vi "NavbalLabVIEW(15-5-28.vi"() -> ()   [LabVIEW 2012] (continued)
                    # "4 Planes were available:\n\nRun solver for all combinations of those 4 planes\n\nOrder:\n0) 1-1-1-1\n1) 1-0-1-1\n2) 0-1-1-1\n3) 1-1-0-1\n4) 1-0-0-1\n5) 0-1-0-1\n6) 0-0-1-1"
                    n2196 = for {
                      N: 15 -> [_]
                      tunnel: w2266 -> [w2269]
                      tunnel: w2265 -> [w2268]
                      i -> [w2270]
                      n2197 = case shown="14" w2270 {
                        tunnel: w2269 -> [w2276 w2301 w2322 w2341 w2365 w2373 w2414 w2434 w2457 w2481 w2504 w2530 w2557 w2583 w2644]
                        tunnel: w2268 -> [w2277 w2298 w2316 w2337 w2356 w2374 w2399 w2422 w2441 w2462 w2488 w2512 w2543 w2564 w2593]
                        frame 0, Default {
                          n2198 = local read "Max Iteration Count"() -> (w2275:dbl)
                          n2199 = local read "Iterative Solution?"() -> (w2274:bool)
                          n2200 = call "SolutionCalculator (SubVI) (2).vi"("Iterative?"=w2274, "Max Iteration Count"=w2275, "Base Run (matrix)"=w2277, "Response Coefficients"=w2276) -> ("Correction Phase (radians)"=w2273:T3, "RMS Residual"=w2271:dbl, "Correction Mag"=w2272:T3)  [unwired: 1 out]
                          n2201 = call-poly <vilib>:"Multiply.vi"("Real Scalar c"=180.0 ("y"), "Real Matrix A"=w2273) -> ("A * c"=w2281:T3)
                          n2202 = Divide(x=w2281, y=3.141592653589793) -> (x/y=w2279:T3)
                          n2203 = Round To Nearest(number=w2279) -> (nearest integer value=w2278:T3)
                          n2204 = local write "Final Mag 0"(w2272) -> ()
                          n2205 = local write "Resid 0"(w2271) -> ()
                          n2206 = local write "Final Phase 0"(w2278) -> ()
                        }
                        frame 1 {
                          w2302 = 2  # Plane Number
                          n2207 = Decrement(x=w2302) -> (x-1=w2299:i32)
                          n2208 = Delete From Array(array=w2301, index (col)=w2299) -> (array with subset deleted=w2297:cdb[][])  [unwired: 2 in, 1 out]
                          n2209 = local read "Max Iteration Count"() -> (w2296:dbl)
                          n2210 = local read "Iterative Solution?"() -> (w2295:bool)
                          n2211 = call "SolutionCalculator (SubVI) (2).vi"("Iterative?"=w2295, "Max Iteration Count"=w2296, "Base Run (matrix)"=w2298, "Response Coefficients"=w2297) -> ("Correction Phase (radians)"=w2293:T3, "RMS Residual"=w2283:dbl, "Correction Mag"=w2294:T3)  [unwired: 1 out]
                          n2212 = call-poly <vilib>:"Polar To Complex.vi"("Argument Q"=w2293, "Modulus r"=w2294) -> ("Complex Matrix r*e^iQ"=w2292:T15)
                          n2213 = Insert Into Array(array=w2292, index (row)=w2299, new element=cdb[] [0.0+0.0i, 0.0+0.0i] ("new element/subarray")) -> (w2284:T15)  [unwired: 1 in]
                          n2214 = call-poly <vilib>:"Complex To Polar.vi"("Complex Matrix r*e^iQ"=w2284) -> ("Modulus r"=w2291:T3, "Argument Q"=w2286:T3)
                          n2215 = call-poly <vilib>:"Multiply.vi"("Real Scalar c"=180.0 ("y"), "Real Matrix A"=w2286) -> ("A * c"=w2288:T3)
                          n2216 = local write "Resid 1"(w2283) -> ()
                          n2217 = Divide(x=w2288, y=3.141592653589793) -> (x/y=w2285:T3)
                          n2218 = Round To Nearest(number=w2285) -> (nearest integer value=w2290:T3)
                          n2219 = local write "Final Mag 1"(w2291) -> ()
                          n2220 = local write "Final Phase 1"(w2290) -> ()
                        }
                        frame 2 {
                          w2319 = 1  # Plane Number
                          n2221 = Decrement(x=w2319) -> (x-1=w2320:i32)
                          n2222 = local read "Max Iteration Count"() -> (w2314:dbl)
                          n2223 = Delete From Array(array=w2322, index (col)=w2320) -> (array with subset deleted=w2315:cdb[][])  [unwired: 2 in, 1 out]
                          n2224 = local read "Iterative Solution?"() -> (w2313:bool)
                          n2225 = call "SolutionCalculator (SubVI) (2).vi"("Iterative?"=w2313, "Max Iteration Count"=w2314, "Base Run (matrix)"=w2316, "Response Coefficients"=w2315) -> ("Correction Phase (radians)"=w2317:T3, "RMS Residual"=w2303:dbl, "Correction Mag"=w2318:T3)  [unwired: 1 out]
                          n2226 = local write "Resid 2"(w2303) -> ()
                          n2227 = call-poly <vilib>:"Polar To Complex.vi"("Argument Q"=w2317, "Modulus r"=w2318) -> ("Complex Matrix r*e^iQ"=w2312:T15)
                          n2228 = Insert Into Array(array=w2312, index (row)=w2320, new element=cdb[] [0.0+0.0i, 0.0+0.0i] ("new element/subarray")) -> (w2304:T15)  [unwired: 1 in]
                          n2229 = call-poly <vilib>:"Complex To Polar.vi"("Complex Matrix r*e^iQ"=w2304) -> ("Modulus r"=w2310:T3, "Argument Q"=w2305:T3)
                          n2230 = call-poly <vilib>:"Multiply.vi"("Real Scalar c"=180.0 ("y"), "Real Matrix A"=w2305) -> ("A * c"=w2308:T3)
                          n2231 = Divide(x=w2308, y=3.141592653589793) -> (x/y=w2306:T3)
                          n2232 = Round To Nearest(number=w2306) -> (nearest integer value=w2311:T3)
                          n2233 = local write "Final Mag  2"(w2310) -> ()
                          n2234 = local write "Final Phase 2"(w2311) -> ()
                        }
                        frame 3 {
                          w2342 = 3  # Plane Number
                          n2235 = Decrement(x=w2342) -> (x-1=w2339:i32)
                          n2236 = Delete From Array(array=w2341, index (col)=w2339) -> (array with subset deleted=w2336:cdb[][])  [unwired: 2 in, 1 out]
                          n2237 = local read "Max Iteration Count"() -> (w2335:dbl)
                          n2238 = local read "Iterative Solution?"() -> (w2334:bool)
                          n2239 = call "SolutionCalculator (SubVI) (2).vi"("Iterative?"=w2334, "Max Iteration Count"=w2335, "Base Run (matrix)"=w2337, "Response Coefficients"=w2336) -> ("Correction Phase (radians)"=w2338:T3, "RMS Residual"=w2323:dbl, "Correction Mag"=w2333:T3)  [unwired: 1 out]
                          n2240 = local write "Resid 3"(w2323) -> ()
                          n2241 = call-poly <vilib>:"Polar To Complex.vi"("Argument Q"=w2338, "Modulus r"=w2333) -> ("Complex Matrix r*e^iQ"=w2324:T15)
                          n2242 = Insert Into Array(array=w2324, index (row)=w2339, new element=cdb[] [0.0+0.0i, 0.0+0.0i] ("new element/subarray")) -> (w2325:T15)  [unwired: 1 in]
                          n2243 = call-poly <vilib>:"Complex To Polar.vi"("Complex Matrix r*e^iQ"=w2325) -> ("Modulus r"=w2326:T3, "Argument Q"=w2328:T3)
                          n2244 = call-poly <vilib>:"Multiply.vi"("Real Scalar c"=180.0 ("y"), "Real Matrix A"=w2328) -> ("A * c"=w2330:T3)
                          n2245 = Divide(x=w2330, y=3.141592653589793) -> (x/y=w2327:T3)
                          n2246 = Round To Nearest(number=w2327) -> (nearest integer value=w2332:T3)
                          n2247 = local write "Final Mag 3"(w2326) -> ()
                          n2248 = local write "Final Phase 3"(w2332) -> ()
                        }
                        frame 4 {
                          w2361 = 2  # Plane Number
                          w2366 = 3  # Plane Number
                          n2249 = local read "Max Iteration Count"() -> (w2354:dbl)
                          n2250 = local read "Iterative Solution?"() -> (w2353:bool)
                          n2251 = Decrement(x=w2366) -> (x-1=w2363:i32)
                          n2252 = Decrement(x=w2361) -> (x-1=w2360:i32)
                          n2253 = Delete From Array(array=w2365, index (col)=w2363) -> (array with subset deleted=w2362:cdb[][])  [unwired: 2 in, 1 out]
                          n2254 = Delete From Array(array=w2362, index (col)=w2360) -> (array with subset deleted=w2355:cdb[][])  [unwired: 2 in, 1 out]
                          n2255 = call "SolutionCalculator (SubVI) (2).vi"("Iterative?"=w2353, "Max Iteration Count"=w2354, "Base Run (matrix)"=w2356, "Response Coefficients"=w2355) -> ("Correction Phase (radians)"=w2357:T3, "RMS Residual"=w2343:dbl, "Correction Mag"=w2358:T3)  [unwired: 1 out]
                          n2256 = call-poly <vilib>:"Polar To Complex.vi"("Argument Q"=w2357, "Modulus r"=w2358) -> ("Complex Matrix r*e^iQ"=w2352:T15)
                          n2257 = Insert Into Array(array=w2352, index (row)=1 ("y"), new element=cdb[][] [[0.0+0.0i, 0.0+0.0i], [0.0+0.0i, 0.0+0.0i]] ("new element/subarray")) -> (w2344:T15)  [unwired: 1 in]
                          n2258 = call-poly <vilib>:"Complex To Polar.vi"("Complex Matrix r*e^iQ"=w2344) -> ("Modulus r"=w2350:T3, "Argument Q"=w2346:T3)
                          n2259 = call-poly <vilib>:"Multiply.vi"("Real Scalar c"=180.0 ("y"), "Real Matrix A"=w2346) -> ("A * c"=w2348:T3)
                          n2260 = Divide(x=w2348, y=3.141592653589793) -> (x/y=w2345:T3)
                          n2261 = Round To Nearest(number=w2345) -> (nearest integer value=w2351:T3)
                          n2262 = local write "Final Mag 4"(w2350) -> ()
                          n2263 = local write "Final Phase 4"(w2351) -> ()
                          n2264 = local write "Resid 4"(w2343) -> ()
                        }
                        frame 5 {
                          w2389 = 1  # Plane Number
                          w2392 = 3  # Plane Number
                          n2265 = local read "Max Iteration Count"() -> (w2371:dbl)
                          n2266 = local read "Iterative Solution?"() -> (w2369:bool)
                          n2267 = Decrement(x=w2392) -> (x-1=w2391:i32)
                          n2268 = Decrement(x=w2389) -> (x-1=w2388:i32)
                          n2269 = Delete From Array(array=w2373, index (col)=w2391) -> (array with subset deleted=w2390:cdb[][])  [unwired: 2 in, 1 out]
                          n2270 = Delete From Array(array=w2390, index (col)=w2388) -> (array with subset deleted=w2370:cdb[][])  [unwired: 2 in, 1 out]
                          n2271 = call "SolutionCalculator (SubVI) (2).vi"("Iterative?"=w2369, "Max Iteration Count"=w2371, "Base Run (matrix)"=w2374, "Response Coefficients"=w2370) -> ("Correction Phase (radians)"=w2375:T3, "RMS Residual"=w2367:dbl, "Correction Mag"=w2376:T3)  [unwired: 1 out]
                          n2272 = call-poly <vilib>:"Polar To Complex.vi"("Argument Q"=w2375, "Modulus r"=w2376) -> ("Complex Matrix r*e^iQ"=w2372:T15)
                          n2273 = local write "Resid 5"(w2367) -> ()
                          n2274 = Insert Into Array(array=w2372, index (row)=1, new element=cdb[] [0.0+0.0i, 0.0+0.0i] ("new element/subarray")) -> (w2385:T15)  [unwired: 1 in]
                          n2275 = Build Array (concatenate)(T15 [[0.0+0.0i]] ("array"), w2385) -> (w2368:T15)
                          n2276 = call-poly <vilib>:"Complex To Polar.vi"("Complex Matrix r*e^iQ"=w2368) -> ("Modulus r"=w2377:T3, "Argument Q"=w2380:T3)
                          n2277 = call-poly <vilib>:"Multiply.vi"("Real Scalar c"=180.0 ("y"), "Real Matrix A"=w2380) -> ("A * c"=w2382:T3)
                          n2278 = Divide(x=w2382, y=3.141592653589793) -> (x/y=w2379:T3)
                          n2279 = Round To Nearest(number=w2379) -> (nearest integer value=w2378:T3)
                          n2280 = local write "Final Mag  5"(w2377) -> ()
                          n2281 = local write "Final Phase 5"(w2378) -> ()
                        }
                        frame 6 {
                          w2409 = T15 [[0.0+0.0i]] ("array")
                          w2411 = 1  # Plane Number
                          w2415 = 2  # Plane Number
                          n2282 = local read "Max Iteration Count"() -> (w2397:dbl)
                          n2283 = local read "Iterative Solution?"() -> (w2396:bool)
                          n2284 = Decrement(x=w2415) -> (x-1=w2413:i32)
                          n2285 = Decrement(x=w2411) -> (x-1=w2410:i32)
                          n2286 = Delete From Array(array=w2414, index (col)=w2413) -> (array with subset deleted=w2412:cdb[][])  [unwired: 2 in, 1 out]
                          n2287 = Delete From Array(array=w2412, index (col)=w2410) -> (array with subset deleted=w2398:cdb[][])  [unwired: 2 in, 1 out]
                          n2288 = call "SolutionCalculator (SubVI) (2).vi"("Iterative?"=w2396, "Max Iteration Count"=w2397, "Base Run (matrix)"=w2399, "Response Coefficients"=w2398) -> ("Correction Phase (radians)"=w2400:T3, "RMS Residual"=w2393:dbl, "Correction Mag"=w2401:T3)  [unwired: 1 out]
                          n2289 = local write "Resid 6"(w2393) -> ()
                          n2290 = call-poly <vilib>:"Polar To Complex.vi"("Argument Q"=w2400, "Modulus r"=w2401) -> ("Complex Matrix r*e^iQ"=w2395:T15)
                          n2291 = Build Array (concatenate)(w2409, w2409, w2395) -> (w2394:T15)
                          n2292 = call-poly <vilib>:"Complex To Polar.vi"("Complex Matrix r*e^iQ"=w2394) -> ("Modulus r"=w2402:T3, "Argument Q"=w2405:T3)
                          n2293 = call-poly <vilib>:"Multiply.vi"("Real Scalar c"=180.0 ("y"), "Real Matrix A"=w2405) -> ("A * c"=w2407:T3)
                          n2294 = Divide(x=w2407, y=3.141592653589793) -> (x/y=w2404:T3)
                          n2295 = Round To Nearest(number=w2404) -> (nearest integer value=w2403:T3)
                          n2296 = local write "Final Phase 6"(w2403) -> ()
                          n2297 = local write "Final Mag  6"(w2402) -> ()
                        }
                        frame 7 {
                          w2435 = 4  # Plane Number
                          n2298 = local read "Max Iteration Count"() -> (w2420:dbl)
                          n2299 = local read "Iterative Solution?"() -> (w2419:bool)
                          n2300 = Decrement(x=w2435) -> (x-1=w2433:i32)
                          n2301 = Delete From Array(array=w2434, index (col)=w2433) -> (array with subset deleted=w2421:cdb[][])  [unwired: 2 in, 1 out]
                          n2302 = call "SolutionCalculator (SubVI) (2).vi"("Iterative?"=w2419, "Max Iteration Count"=w2420, "Base Run (matrix)"=w2422, "Response Coefficients"=w2421) -> ("Correction Phase (radians)"=w2423:T3, "RMS Residual"=→"Resid 7":dbl, "Correction Mag"=w2424:T3)  [unwired: 1 out]
                          n2303 = call-poly <vilib>:"Polar To Complex.vi"("Argument Q"=w2423, "Modulus r"=w2424) -> ("Complex Matrix r*e^iQ"=w2418:T15)
                          n2304 = Build Array (concatenate)(w2418, T15 [[0.0+0.0i]] ("array")) -> (w2417:T15)
                          n2305 = call-poly <vilib>:"Complex To Polar.vi"("Complex Matrix r*e^iQ"=w2417) -> ("Modulus r"=→"Final Mag  7":T3, "Argument Q"=w2427:T3)
                          n2306 = call-poly <vilib>:"Multiply.vi"("Real Scalar c"=180.0 ("y"), "Real Matrix A"=w2427) -> ("A * c"=w2429:T3)
                          n2307 = Divide(x=w2429, y=3.141592653589793) -> (x/y=w2426:T3)
                          n2308 = Round To Nearest(number=w2426) -> (nearest integer value=→"Final Phase 7":T3)
                        }
                        frame 8 {
                          w2452 = T15 [[0.0+0.0i]] ("array")
                          w2454 = 1  # Plane Number
                          w2458 = 4  # Plane Number
                          n2309 = local read "Max Iteration Count"() -> (w2440:dbl)
                          n2310 = local read "Iterative Solution?"() -> (w2439:bool)
                          n2311 = Decrement(x=w2458) -> (x-1=w2456:i32)
                          n2312 = Decrement(x=w2454) -> (x-1=w2453:i32)
                          n2313 = Delete From Array(array=w2457, index (col)=w2456) -> (array with subset deleted=w2455:cdb[][])  [unwired: 2 in, 1 out]
                          n2314 = Delete From Array(array=w2455, index (col)=w2453) -> (array with subset deleted=w2442:cdb[][])  [unwired: 2 in, 1 out]
                          n2315 = call "SolutionCalculator (SubVI) (2).vi"("Iterative?"=w2439, "Max Iteration Count"=w2440, "Base Run (matrix)"=w2441, "Response Coefficients"=w2442) -> ("Correction Phase (radians)"=w2443:T3, "RMS Residual"=→"Resid 8":dbl, "Correction Mag"=w2444:T3)  [unwired: 1 out]
                          n2316 = call-poly <vilib>:"Polar To Complex.vi"("Argument Q"=w2443, "Modulus r"=w2444) -> ("Complex Matrix r*e^iQ"=w2438:T15)
                          n2317 = Build Array (concatenate)(w2452, w2438, w2452) -> (w2437:T15)
                          n2318 = call-poly <vilib>:"Complex To Polar.vi"("Complex Matrix r*e^iQ"=w2437) -> ("Modulus r"=→"Final Mag 8":T3, "Argument Q"=w2446:T3)
                          n2319 = call-poly <vilib>:"Multiply.vi"("Real Scalar c"=180.0 ("y"), "Real Matrix A"=w2446) -> ("A * c"=w2448:T3)
                          n2320 = Divide(x=w2448, y=3.141592653589793) -> (x/y=w2445:T3)
                          n2321 = Round To Nearest(number=w2445) -> (nearest integer value=→"Final Phase 8":T3)
                        }
                        frame 9 {
                          w2478 = 2  # Plane Number
                          w2482 = 4  # Plane Number
                          n2322 = Decrement(x=w2482) -> (x-1=w2480:i32)
                          n2323 = Decrement(x=w2478) -> (x-1=w2477:i32)
                          n2324 = Delete From Array(array=w2481, index (col)=w2480) -> (array with subset deleted=w2479:cdb[][])  [unwired: 2 in, 1 out]
                          n2325 = Delete From Array(array=w2479, index (col)=w2477) -> (array with subset deleted=w2463:cdb[][])  [unwired: 2 in, 1 out]
                          n2326 = call "SolutionCalculator (SubVI) (2).vi"("Base Run (matrix)"=w2462, "Response Coefficients"=w2463) -> ("Correction Phase (radians)"=w2464:T3, "RMS Residual"=→"Resid 9":dbl, "Correction Mag"=w2465:T3)  [unwired: 2 in, 1 out]
                          n2327 = call-poly <vilib>:"Polar To Complex.vi"("Argument Q"=w2464, "Modulus r"=w2465) -> ("Complex Matrix r*e^iQ"=w2461:T15)
                          n2328 = Insert Into Array(array=w2461, index (row)=1, new element=cdb[] [0.0+0.0i, 0.0+0.0i] ("new element/subarray")) -> (w2473:T15)  [unwired: 1 in]
                          n2329 = Build Array (concatenate)(w2473, T15 [[0.0+0.0i]] ("array")) -> (w2460:T15)
                          n2330 = call-poly <vilib>:"Complex To Polar.vi"("Complex Matrix r*e^iQ"=w2460) -> ("Modulus r"=→"Final Mag 9":T3, "Argument Q"=w2467:T3)
                          n2331 = call-poly <vilib>:"Multiply.vi"("Real Scalar c"=180.0 ("y"), "Real Matrix A"=w2467) -> ("A * c"=w2469:T3)
                          n2332 = Divide(x=w2469, y=3.141592653589793) -> (x/y=w2466:T3)
                          n2333 = Round To Nearest(number=w2466) -> (nearest integer value=→"Final Phase 9":T3)
                        }
                        frame 10 {
                          w2499 = T15 [[0.0+0.0i]] ("array")
                          w2501 = 3  # Plane Number
                          w2505 = 4  # Plane Number
                          n2334 = Decrement(x=w2505) -> (x-1=w2503:i32)
                          n2335 = local read "Max Iteration Count"() -> (w2487:dbl)
                          n2336 = local read "Iterative Solution?"() -> (w2486:bool)
                          n2337 = Decrement(x=w2501) -> (x-1=w2500:i32)
                          n2338 = Delete From Array(array=w2504, index (col)=w2503) -> (array with subset deleted=w2502:cdb[][])  [unwired: 2 in, 1 out]
                          n2339 = Delete From Array(array=w2502, index (col)=w2500) -> (array with subset deleted=w2489:cdb[][])  [unwired: 2 in, 1 out]
                          n2340 = call "SolutionCalculator (SubVI) (2).vi"("Iterative?"=w2486, "Max Iteration Count"=w2487, "Base Run (matrix)"=w2488, "Response Coefficients"=w2489) -> ("Correction Phase (radians)"=w2490:T3, "RMS Residual"=→"Resid 10":dbl, "Correction Mag"=w2491:T3)  [unwired: 1 out]
                          n2341 = call-poly <vilib>:"Polar To Complex.vi"("Argument Q"=w2490, "Modulus r"=w2491) -> ("Complex Matrix r*e^iQ"=w2485:T15)
                          n2342 = Build Array (concatenate)(w2485, w2499, w2499) -> (w2484:T15)
                          n2343 = call-poly <vilib>:"Complex To Polar.vi"("Complex Matrix r*e^iQ"=w2484) -> ("Modulus r"=→"Final Mag 10":T3, "Argument Q"=w2493:T3)
                          n2344 = call-poly <vilib>:"Multiply.vi"("Real Scalar c"=180.0 ("y"), "Real Matrix A"=w2493) -> ("A * c"=w2495:T3)
                          n2345 = Divide(x=w2495, y=3.141592653589793) -> (x/y=w2492:T3)
                          n2346 = Round To Nearest(number=w2492) -> (nearest integer value=→"Final Phase 10":T3)
                        }
                        frame 11 {
                          w2523 = 2  # Plane Number
                          w2526 = T15 [[0.0+0.0i]] ("array")
                          w2522 = 3  # Plane Number
                          w2531 = 4  # Plane Number
                          n2347 = local read "Max Iteration Count"() -> (w2508:dbl)
                          n2348 = local read "Iterative Solution?"() -> (w2507:bool)
                          n2349 = Decrement(x=w2531) -> (x-1=w2529:i32)
                          n2350 = Decrement(x=w2522) -> (x-1=w2527:i32)
                          n2351 = Decrement(x=w2523) -> (x-1=w2524:i32)
                          n2352 = Delete From Array(array=w2530, index (col)=w2529) -> (array with subset deleted=w2528:cdb[][])  [unwired: 2 in, 1 out]
                          n2353 = Delete From Array(array=w2528, index (col)=w2527) -> (array with subset deleted=w2525:cdb[][])  [unwired: 2 in, 1 out]
                          n2354 = Delete From Array(array=w2525, index (col)=w2524) -> (array with subset deleted=w2511:cdb[][])  [unwired: 2 in, 1 out]
                          n2355 = call "SolutionCalculator (SubVI) (2).vi"("Iterative?"=w2507, "Max Iteration Count"=w2508, "Base Run (matrix)"=w2512, "Response Coefficients"=w2511) -> ("Correction Phase (radians)"=w2513:T3, "RMS Residual"=→"Resid 11":dbl, "Correction Mag"=w2514:T3)  [unwired: 1 out]
                          n2356 = call-poly <vilib>:"Polar To Complex.vi"("Argument Q"=w2513, "Modulus r"=w2514) -> ("Complex Matrix r*e^iQ"=w2510:T15)
                          n2357 = Build Array (concatenate)(w2510, w2526, w2526, w2526) -> (w2509:T15)
                          n2358 = call-poly <vilib>:"Complex To Polar.vi"("Complex Matrix r*e^iQ"=w2509) -> ("Modulus r"=→"Final Mag 11":T3, "Argument Q"=w2516:T3)
                          n2359 = call-poly <vilib>:"Multiply.vi"("Real Scalar c"=180.0 ("y"), "Real Matrix A"=w2516) -> ("A * c"=w2518:T3)
                          n2360 = Divide(x=w2518, y=3.141592653589793) -> (x/y=w2515:T3)
                          n2361 = Round To Nearest(number=w2515) -> (nearest integer value=→"Final Phase 11":T3)
                        }
                        frame 12 {
                          w2534 = 1  # Plane Number
                          w2554 = T15 [[0.0+0.0i]] ("array")
                          w2536 = 3  # Plane Number
                          w2538 = 4  # Plane Number
                          n2362 = Decrement(x=w2538) -> (x-1=w2537:i32)
                          n2363 = Decrement(x=w2536) -> (x-1=w2535:i32)
                          n2364 = Decrement(x=w2534) -> (x-1=w2533:i32)
                          n2365 = local read "Max Iteration Count"() -> (w2542:dbl)
                          n2366 = local read "Iterative Solution?"() -> (w2541:bool)
                          n2367 = Delete From Array(array=w2557, index (col)=w2537) -> (array with subset deleted=w2556:cdb[][])  [unwired: 2 in, 1 out]
                          n2368 = Delete From Array(array=w2556, index (col)=w2535) -> (array with subset deleted=w2555:cdb[][])  [unwired: 2 in, 1 out]
                          n2369 = Delete From Array(array=w2555, index (col)=w2533) -> (array with subset deleted=w2544:cdb[][])  [unwired: 2 in, 1 out]
                          n2370 = call "SolutionCalculator (SubVI) (2).vi"("Iterative?"=w2541, "Max Iteration Count"=w2542, "Base Run (matrix)"=w2543, "Response Coefficients"=w2544) -> ("Correction Phase (radians)"=w2545:T3, "RMS Residual"=→"Resid 12":dbl, "Correction Mag"=w2546:T3)  [unwired: 1 out]
                          n2371 = call-poly <vilib>:"Polar To Complex.vi"("Argument Q"=w2545, "Modulus r"=w2546) -> ("Complex Matrix r*e^iQ"=w2540:T15)
                          n2372 = Build Array (concatenate)(w2554, w2540, w2554, w2554) -> (w2539:T15)
                          n2373 = call-poly <vilib>:"Complex To Polar.vi"("Complex Matrix r*e^iQ"=w2539) -> ("Modulus r"=→"Final Mag 12":T3, "Argument Q"=w2548:T3)
                          n2374 = call-poly <vilib>:"Multiply.vi"("Real Scalar c"=180.0 ("y"), "Real Matrix A"=w2548) -> ("A * c"=w2550:T3)
                          n2375 = Divide(x=w2550, y=3.141592653589793) -> (x/y=w2547:T3)
                          n2376 = Round To Nearest(number=w2547) -> (nearest integer value=→"Final Phase 12":T3)
                        }
                        frame 13 {
                          w2578 = 1  # Plane Number
                          w2580 = T15 [[0.0+0.0i]] ("array")
                          w2577 = 2  # Plane Number
                          w2576 = 4  # Plane Number
                          n2377 = Decrement(x=w2576) -> (x-1=w2579:i32)
                          n2378 = Decrement(x=w2577) -> (x-1=w2575:i32)
                          n2379 = Decrement(x=w2578) -> (x-1=w2574:i32)
                          n2380 = Delete From Array(array=w2583, index (col)=w2579) -> (array with subset deleted=w2582:cdb[][])  [unwired: 2 in, 1 out]
                          n2381 = Delete From Array(array=w2582, index (col)=w2575) -> (array with subset deleted=w2581:cdb[][])  [unwired: 2 in, 1 out]
                          n2382 = local read "Max Iteration Count"() -> (w2562:dbl)
                          n2383 = local read "Iterative Solution?"() -> (w2561:bool)
                          n2384 = Delete From Array(array=w2581, index (col)=w2574) -> (array with subset deleted=w2563:cdb[][])  [unwired: 2 in, 1 out]
                          n2385 = call "SolutionCalculator (SubVI) (2).vi"("Iterative?"=w2561, "Max Iteration Count"=w2562, "Base Run (matrix)"=w2564, "Response Coefficients"=w2563) -> ("Correction Phase (radians)"=w2565:T3, "RMS Residual"=→"Resid 13":dbl, "Correction Mag"=w2566:T3)  [unwired: 1 out]
                          n2386 = call-poly <vilib>:"Polar To Complex.vi"("Argument Q"=w2565, "Modulus r"=w2566) -> ("Complex Matrix r*e^iQ"=w2560:T15)
                          n2387 = Build Array (concatenate)(w2580, w2580, w2560, w2580) -> (w2559:T15)
                          n2388 = call-poly <vilib>:"Complex To Polar.vi"("Complex Matrix r*e^iQ"=w2559) -> ("Modulus r"=→"Final Mag 13":T3, "Argument Q"=w2568:T3)
                          n2389 = call-poly <vilib>:"Multiply.vi"("Real Scalar c"=180.0 ("y"), "Real Matrix A"=w2568) -> ("A * c"=w2570:T3)
                          n2390 = Divide(x=w2570, y=3.141592653589793) -> (x/y=w2567:T3)
                          n2391 = Round To Nearest(number=w2567) -> (nearest integer value=→"Final Phase 13":T3)
                        }
                        frame 14 {
                          w2604 = 1  # Plane Number
                          w2641 = T15 [[0.0+0.0i]] ("array")
                          w2605 = 2  # Plane Number
                          w2606 = 3  # Plane Number
                          n2392 = local read "Max Iteration Count"() -> (w2591:dbl)
                          n2393 = local read "Iterative Solution?"() -> (w2590:bool)
                          n2394 = Decrement(x=w2606) -> (x-1=w2587:i32)
                          n2395 = Decrement(x=w2605) -> (x-1=w2602:i32)
                          n2396 = Decrement(x=w2604) -> (x-1=w2603:i32)
                          n2397 = Delete From Array(array=w2644, index (col)=w2587) -> (array with subset deleted=w2643:cdb[][])  [unwired: 2 in, 1 out]
                          n2398 = Delete From Array(array=w2643, index (col)=w2602) -> (array with subset deleted=w2642:cdb[][])  [unwired: 2 in, 1 out]
                          n2399 = Delete From Array(array=w2642, index (col)=w2603) -> (array with subset deleted=w2592:cdb[][])  [unwired: 2 in, 1 out]
                          n2400 = call "SolutionCalculator (SubVI) (2).vi"("Iterative?"=w2590, "Max Iteration Count"=w2591, "Base Run (matrix)"=w2593, "Response Coefficients"=w2592) -> ("Correction Phase (radians)"=w2594:T3, "RMS Residual"=w2586:dbl, "Correction Mag"=w2595:T3)  [unwired: 1 out]
                          "Resid 14" <- w2586
                          n2401 = call-poly <vilib>:"Polar To Complex.vi"("Argument Q"=w2594, "Modulus r"=w2595) -> ("Complex Matrix r*e^iQ"=w2589:T15)
                          n2402 = Build Array (concatenate)(w2641, w2641, w2641, w2589) -> (w2588:T15)
                          n2403 = local read "Final Mag 0"() -> (w2620:T3)
                          n2404 = local read "Final Mag  2"() -> (w2617:T3)
                          n2405 = local read "Final Mag  5"() -> (w2614:T3)
                          n2406 = local read "Final Mag  6"() -> (w2624:T3)
                          n2407 = local read "Final Mag  7"() -> (w2625:T3)
                          n2408 = local read "Final Mag 9"() -> (w2627:T3)
                          n2409 = local read "Final Mag 1"() -> (w2621:T3)
                          n2410 = local read "Final Mag 3"() -> (w2616:T3)
                          n2411 = local read "Final Mag 4"() -> (w2615:T3)
                          n2412 = local read "Final Mag 8"() -> (w2626:T3)
                          n2413 = local read "Final Mag 10"() -> (w2628:T3)
                          n2414 = local read "Final Mag 11"() -> (w2629:T3)
                          n2415 = local read "Final Mag 12"() -> (w2630:T3)
                          n2416 = local read "Final Mag 13"() -> (w2631:T3)
                          n2417 = call-poly <vilib>:"Complex To Polar.vi"("Complex Matrix r*e^iQ"=w2588) -> ("Modulus r"=w2609:T3, "Argument Q"=w2597:T3)
                          "Final Mag 14" <- w2609
                          n2418 = call-poly <vilib>:"Multiply.vi"("Real Scalar c"=180.0 ("y"), "Real Matrix A"=w2597) -> ("A * c"=w2599:T3)
                          n2419 = Divide(x=w2599, y=3.141592653589793) -> (x/y=w2596:T3)
                          n2420 = Build Array (concatenate)(w2620, w2621, w2617, w2616, w2615, w2614, w2624, w2625, w2626, w2627, w2628, w2629, w2630, w2631, w2609) -> (w2608:T3)
                          n2421 = Round To Nearest(number=w2596) -> (nearest integer value=→"Final Phase 14":T3)
                          n2422 = local read "Resid 0"() -> (w2618:dbl)
                          n2423 = local read "Resid 1"() -> (w2619:dbl)
                          n2424 = local read "Resid 2"() -> (w2613:dbl)
                          n2425 = local read "Resid 3"() -> (w2612:dbl)
                          n2426 = local read "Resid 4"() -> (w2611:dbl)
                          n2427 = local read "Resid 5"() -> (w2610:dbl)
                          n2428 = local read "Resid 6"() -> (w2632:dbl)
                          n2429 = local read "Resid 7"() -> (w2633:dbl)
                          n2430 = local read "Resid 8"() -> (w2634:dbl)
                          n2431 = local read "Resid 9"() -> (w2635:dbl)
                          n2432 = local read "Resid 10"() -> (w2636:dbl)
                          n2433 = local read "Resid 11"() -> (w2637:dbl)
                          n2434 = local read "Resid 12"() -> (w2638:dbl)
                          n2435 = local read "Resid 13"() -> (w2639:dbl)
                          n2436 = Transpose 2D Array(2D array=w2608) -> (transposed array=w2607:T3)
                          n2437 = Build Array(w2618, w2619, w2613, w2612, w2611, w2610, w2632, w2633, w2634, w2635, w2636, w2637, w2638, w2639, w2586) -> (w2640:T3)
                          n2438 = Build Array (concatenate)(w2607, w2640) -> (w2623:T3)
                          n2439 = Number To Fractional String(number=w2623, precision (6)=i16 3) -> (F-format string=w2585:string[][])  [unwired: 2 in]
                          n2440 = for {
                            tunnel: w2585 -> [w2646] mode=indexing
                            tunnel: [w2645] -> w2584 mode=indexing
                            n2441 = for {
                              tunnel: w2646 -> [w2647] mode=indexing
                              tunnel: [w2648] -> w2645 mode=indexing
                              n2442 = Equal?(x="0.000", y=w2647) -> (x = y?=w2649:bool)
                              n2443 = case shown="False" w2649 {
                                tunnel: [w2651 ""] -> w2648
                                tunnel: w2647 -> [w2651 _]
                                frame False {
                                }
                                frame True {
                                }
                              }
                            }
                          }
                          n2444 = property on="Solution Options" class="MCListbox (strict)"("ItemNames"=w2584) -> ()  [unwired: 2 in, 2 out]
                        }
                      }
                    }
                  }
                }
              }
            }
          }
        }
        n2445 = case "Begin Weight Splitting Procedure:\n\nProcess is to use a binary search algorithm to most closely match the  \"ideal vector\". If we use brute force, solution\ncomplexity is about N^2, or about 2e8 combinations, versus the binary search, which is NlogN, or 6e4 combinations \n\nProcess also checks to see if current hole is occupied in that plane, and will alter vector combinations which use that hole\nso that they are not selected as the best combination" shown="True" "Split Weights" {
          tunnel: "Degrees" -> [_ w2657]
          tunnel: "Ideal Weight" -> [_ w2659]
          tunnel: w634 -> [_ w2658]
          frame False {
            # "Useful to check here, but I didnt store any code inside.\n\n-Belding"
          }
          frame True {
            w2660 = u32 2771455
            # "Generate ideal  complex vector"
            # "4 planes"
            # "get number of \nholes"
            n2446 = Divide(x=w2657, y=180.0 ("x")) -> (x/y=w2664:T3)
            n2447 = for "Clear Prediction highlights" {
              N: 50 -> [_]
              i -> [w2672]
              n2448 = Bundle(w2672, "Column"=3) -> (w2671:cluster{i32, "Column":i32})  [unwired: 1 in]
              n2449 = property on="Prediction Results" class="MCListbox (strict)"("ActiveCell"=w2671) -> ()  [unwired: 2 in, 2 out]
              n2450 = property on="Prediction Results" class="MCListbox (strict)"("CellBG"=u32 16777215) -> ()  [unwired: 2 in, 2 out]
            }
            n2451 = property on="Aft Turbine Balance Plane Split Options" class="MCListbox (strict)"("SelColor"=w2660) -> ()  [unwired: 2 in, 2 out]
            n2452 = property on="Fwd Turbine Balance Plane Split Options" class="MCListbox (strict)"("SelColor"=w2660) -> ()  [unwired: 2 in, 2 out]
            n2453 = case shown="\"Port\"" w2658 {
              tunnel: ["Existing Plane Wts Stbd" "Existing Plane Wts Port"] -> w2653
              frame "Starboard", Default {
              }
              frame "Port" {
              }
            }
            n2454 = property on="Aft Generator Balance Plane Split Options" class="MCListbox (strict)"("SelColor"=w2660) -> ()  [unwired: 2 in, 2 out]
            n2455 = property on="Fwd Generator Balance Plane Split Options" class="MCListbox (strict)"("SelColor"=w2660) -> ()  [unwired: 2 in, 2 out]
            n2456 = call-poly <vilib>:"Multiply.vi"("Real Matrix A"=w2664, "Real Scalar c"=3.141592653589793) -> ("c * A"=w2665:T3)
            n2457 = call-poly <vilib>:"Multiply.vi"("Real Matrix A"="Divisions in\nEach Plane", "Real Scalar c"="Holes/Division") -> ("c * A"=w2662:T3)
            n2458 = call-poly <vilib>:"Polar To Complex.vi"("Argument Q"=w2665, "Modulus r"=w2659) -> ("Complex Matrix r*e^iQ"=w2663:T15)
            n2459 = Matrix Size(0:w2659) -> (1:w2668:i32)  [unwired: 1 out]
            n2460 = for {
              N: w2668 -> [_]
              tunnel: w2659 -> [w2700] mode=indexing
              tunnel: w2663 -> [w2696] mode=indexing
              tunnel: w2662 -> [w2697] mode=indexing
              tunnel: w2657 -> [w2698] mode=indexing
              tunnel: "Divisions in\nEach Plane" -> [w2694] mode=indexing
              tunnel: [w2689] -> w2654 mode=indexing
              tunnel: w2653 -> [w2686]
              i -> [w2688]
              # "Places data into the listbox of split options"
              n2461 = Index Array(array=w2700, index=0) -> (element=w2676:dbl)
              n2462 = Not Equal To 0?(x=w2676) -> (x != 0?=w2675:bool)
              n2463 = case shown="True" w2675 {
                tunnel: [w2707 w2803] -> w2701
                tunnel: [w2707 w2802] -> w2699
                tunnel: w2698 -> [_ w2800]
                tunnel: w2697 -> [_ w2799]
                tunnel: w2696 -> [_ w2787]
                tunnel: [w2707 w2783] -> w2695
                tunnel: w2694 -> [_ w2782]
                tunnel: [cdb 0.0+0.0i w2781] -> w2693
                tunnel: [w2702 w2776] -> w2692
                tunnel: [0.0 w2773] -> w2691
                tunnel: [cdb 0.0+0.0i w2749] -> w2689
                tunnel: w2688 -> [_ w2746]
                tunnel: [0 ("Holes/Division") w2745] -> w2687
                tunnel: w2686 -> [_ w2744]
                tunnel: [bool[][] [] w2743] -> w2685
                tunnel: [cdb 0.0+0.0i w2741] -> w2684
                tunnel: [w2707 w2735] -> w2683
                tunnel: [0.0 ("Closest Angle 1") w2728] -> w2682
                tunnel: [w2707 w2727] -> w2681
                tunnel: [w2702 w2720] -> w2680
                tunnel: [w2702 w2716] -> w2679
                tunnel: [w2707 w2715] -> w2678
                tunnel: [cdb 0.0+0.0i w2713] -> w2677
                tunnel: w2676 -> [_ w2712]
                frame False {
                  w2702 = 0.0 ("Closest Weight 2")
                  w2707 = 0.0
                }
                frame True {
                  w2779 = 360.0 ("x")
                  # "Replace angles in the array that are \nunavailable with the previous angle.\nThus, the binary search algorithm will\navoid those possibilities"
                  # "Generate array of possible angles"
                  # "Conduct binary search operation to find\nclosest option to the split"
                  # "Percent Accuracy of \n2 mass split"
                  # "percent Accuracy of 1 mass"
                  # "# holes"
                  # "format phase in both degrees and hole location"
                  n2464 = Index Array(array=w2799, index=0) -> (element=w2750:dbl)
                  n2465 = Index Array(array=w2787, index=0) -> (element=w2751:cdb)
                  n2466 = Divide(x=360.0, y=w2750) -> (x/y=w2796:dbl)
                  n2467 = Index Array(array=w2782, index=0) -> (element=w2771:dbl)
                  n2468 = for {
                    N: w2750 -> [_]
                    shift-right: [w2828] -> w2748
                    shift-left: dbl[] [] -> [w2831]
                    tunnel: w2796 -> [w2832]
                    i -> [w2830]
                    n2469 = Multiply(x=w2832, y=w2830) -> (x*y=w2829:dbl)
                    n2470 = Insert Into Array(array=w2831, index=w2830, new element=w2829) -> (w2828:dbl[])
                  }
                  n2471 = case shown="0, Default" w2746 {
                    tunnel: [w2833 w2834 w2835 w2836] -> w2714
                    frame 0, Default {
                      n2472 = local read "AT Weights"() -> (w2833:dbl[])
                    }
                    frame 1 {
                      n2473 = local read "FT Weights"() -> (w2834:dbl[])
                    }
                    frame 2 {
                      n2474 = local read "AG Weights"() -> (w2835:dbl[])
                    }
                    frame 3 {
                      n2475 = local read "FG Weights"() -> (w2836:dbl[])
                    }
                  }
                  n2476 = Index Array(array=w2744, index (col)=w2746) -> (element=w2739:dbl[])  [unwired: 1 in]
                  n2477 = Index Array(array=w2800, index=0) -> (element=w2780:dbl)
                  n2478 = case shown="False" "Avoid Occupancies" {
                    tunnel: w2748 -> [w2806 w2808]
                    tunnel: [w2806 w2809] -> w2734
                    tunnel: w2739 -> [_ w2810]
                    tunnel: w2739 -> [_ w2807]
                    tunnel: [dbl[] [] ("Existing Plane Wts Port") w2807] -> w2719
                    frame False {
                    }
                    frame True {
                      n2479 = for {
                        tunnel: w2810 -> [w2813] mode=indexing
                        shift-right: [w2815] -> w2809
                        shift-left: w2808 -> [w2814]
                        i -> [w2816]
                        n2480 = Equal?(x=w2813, y=-1.0) -> (x = y?=w2811:bool)
                        n2481 = Decrement(x=w2816) -> (x-1=w2817:i32)
                        n2482 = case shown="True" w2811 {
                          tunnel: w2814 -> [w2818 w2819]
                          tunnel: w2817 -> [_ w2823]
                          tunnel: w2816 -> [_ w2822]
                          tunnel: [w2818 w2820] -> w2815
                          frame False {
                          }
                          frame True {
                            n2483 = Index Array(array=w2819, index=w2823) -> (element=w2821:dbl)
                            n2484 = Replace Array Subset(array=w2819, new element=w2821, index=w2822) -> (w2820:dbl[])
                          }
                        }
                      }
                    }
                  }
                  n2485 = case shown="3" w2746 {
                    tunnel: [w2824 w2825 w2826 w2827] -> w2740
                    frame 0, Default {
                      n2486 = local read "AT Exceptions"() -> (w2824:csg[])
                    }
                    frame 1 {
                      n2487 = local read "FT Exceptions"() -> (w2825:csg[])
                    }
                    frame 2 {
                      n2488 = local read "AG Exceptions"() -> (w2826:csg[])
                    }
                    frame 3 {
                      n2489 = local read "FG Exceptions"() -> (w2827:csg[])
                    }
                  }
                  n2490 = Array Size(array=w2734) -> (size(s)=w2717:i32)
                  n2491 = call "BinarySearch2.vi"("ExistingWts 1D Array"=w2719, "Exception List"=w2740, "Desired Angle (degrees)"=w2780, "Desired Weight"=w2712, "Angles 1D Array"=w2734, "Weights 1D Array"=w2714) -> ("Closest Angle 2"=w2716:dbl, "Closest Weight 2"=w2720:dbl, "Closest Angle 1"=w2728:dbl, "Closest Weight 1"=w2727:dbl)  [unwired: 2 in]
                  n2492 = call "BinarySearch1.vi"("ExistingWts 1D Array"=w2719, "Desired Angle (degrees)"=w2780, "Desired Weight"=w2712, "Angles 1D Array"=w2734, "Weights 1D Array"=w2714) -> ("Closest Angle 1"=w2735:dbl, "Closest Weight 1"=w2715:dbl)  [unwired: 5 in]
                  n2493 = Divide(x=w2716, y=360.0) -> (x/y=w2723:dbl)
                  n2494 = Multiply(x=w2717, y=w2723) -> (x*y=w2722:dbl)
                  n2495 = Index Array(array=w2719, index=w2722) -> (element=w2721:dbl)
                  n2496 = Divide(x=w2728, y=360.0) -> (x/y=w2730:dbl)
                  n2497 = Divide(x=w2735, y=360.0) -> (x/y=w2737:dbl)
                  n2498 = Subtract(x=w2720, y=w2721) -> (x-y=w2718:dbl)
                  n2499 = Multiply(x=w2717, y=w2730) -> (x*y=w2731:dbl)
                  n2500 = Multiply(x=w2717, y=w2737) -> (x*y=w2736:dbl)
                  n2501 = Index Array(array=w2719, index=w2731) -> (element=w2726:dbl)
                  n2502 = Index Array(array=w2719, index=w2736) -> (element=w2733:dbl)
                  n2503 = Subtract(x=w2727, y=w2726) -> (x-y=w2725:dbl)
                  n2504 = Subtract(x=w2715, y=w2733) -> (x-y=w2732:dbl)
                  n2505 = Multiply(x=w2728, y=3.141592653589793) -> (x*y=w2794:dbl)
                  n2506 = Multiply(x=w2716, y=3.141592653589793) -> (x*y=w2789:dbl)
                  n2507 = Divide(x=w2794, y=180.0 ("x")) -> (x/y=w2792:dbl)
                  n2508 = Divide(x=w2789, y=180.0 ("x")) -> (x/y=w2791:dbl)
                  n2509 = Polar To Complex ("Polar To Complex.vi")(1:w2792, 2:w2725) -> (0:w2713:cdb)
                  n2510 = Polar To Complex ("Polar To Complex.vi")(1:w2791, 2:w2718) -> (0:w2781:cdb)
                  n2511 = Add(x=w2713, y=w2781) -> (x+y=w2749:cdb)
                  n2512 = Subtract(x=w2751, y=w2749) -> (x-y=w2786:cdb)
                  n2513 = Complex To Polar(r * e^(i*theta)=w2751) -> (r=w2784:dbl)  [unwired: 1 out]
                  n2514 = Complex To Polar(r * e^(i*theta)=w2786) -> (r=w2785:dbl)  [unwired: 1 out]
                  n2515 = Multiply(x=w2735, y=3.141592653589793) -> (x*y=w2754:dbl)
                  n2516 = Divide(x=w2785, y=w2784) -> (x/y=w2761:dbl)
                  n2517 = Divide(x=w2754, y=180.0 ("x")) -> (x/y=w2752:dbl)
                  n2518 = Subtract(x=1.0, y=w2761) -> (x-y=w2759:dbl)
                  n2519 = Polar To Complex ("Polar To Complex.vi")(1:w2752, 2:w2732) -> (0:w2741:cdb)
                  n2520 = Multiply(x=w2759, y=100.0) -> (x*y=w2783:dbl)
                  n2521 = Subtract(x=w2741, y=w2751) -> (x-y=w2767:cdb)
                  n2522 = Divide(x=w2735, y=360.0 ("x")) -> (x/y=w2770:dbl)
                  n2523 = Complex To Polar(r * e^(i*theta)=w2767) -> (r=w2766:dbl)  [unwired: 1 out]
                  n2524 = Complex To Polar(r * e^(i*theta)=w2751) -> (r=w2765:dbl)  [unwired: 1 out]
                  n2525 = Multiply(x=w2770, y=w2771) -> (x*y=w2769:dbl)
                  n2526 = Divide(x=w2766, y=w2765) -> (x/y=w2764:dbl)
                  n2527 = Divide(x=w2728, y=w2779) -> (x/y=w2775:dbl)
                  n2528 = Increment(x=w2769) -> (x+1=w2802:dbl)
                  n2529 = Divide(x=w2716, y=w2779) -> (x/y=w2778:dbl)
                  n2530 = Equal?(x=w2744, y=-1.0 ("x")) -> (x = y?=w2743:bool[][])
                  n2531 = Subtract(x=1.0, y=w2764) -> (x-y=w2762:dbl)
                  n2532 = local read "Holes/Division"() -> (w2745:i32)
                  n2533 = Multiply(x=w2778, y=w2771) -> (x*y=w2777:dbl)
                  n2534 = Multiply(x=w2775, y=w2771) -> (x*y=w2774:dbl)
                  n2535 = Increment(x=w2777) -> (x+1=w2776:dbl)
                  n2536 = Increment(x=w2774) -> (x+1=w2773:dbl)
                  n2537 = Multiply(x=w2762, y=100.0) -> (x*y=w2803:dbl)
                }
              }
              n2538 = case shown="0, Default" w2688 {
                tunnel: w2701 -> [w2843 w2921 w3066 w3142]
                tunnel: w2683 -> [w2915 w2991 w3067 w3143]
                tunnel: w2695 -> [w2909 w2985 w3060 w3137]
                tunnel: w2682 -> [w2914 w2990 w3065 w3141]
                tunnel: w2679 -> [w2913 w2989 w3064 w3074]
                tunnel: w2685 -> [w2884 w2960 w3035 w3111]
                tunnel: w2677 -> [w2841 w2918 w2993 w3072]
                tunnel: w2699 -> [w2850 w2927 w3002 w3079]
                tunnel: w2678 -> [w2844 w2922 w2996 w3070]
                tunnel: w2691 -> [w2849 w2926 w3001 w3078]
                tunnel: w2692 -> [w2848 w2925 w3000 w3077]
                tunnel: w2681 -> [w2846 w2923 w2997 w3073]
                tunnel: w2680 -> [w2845 w2920 w2998 w3075]
                tunnel: w2686 -> [w2847 w2924 w2999 w3076]
                tunnel: w2693 -> [w2840 w2917 w2994 w3071]
                tunnel: w2684 -> [w2842 w2919 w2995 w3069]
                tunnel: w2687 -> [w2839 w2916 w2992 w3068]
                frame 0, Default {
                  w2852 = 1 ("dimension size")
                  w2856 = 0 ("disabled index (col)")
                  w2864 = 0 ("disabled index (col)")
                  w2881 = 0 ("disabled index (col)")
                  w2893 = "Occupied!  "
                  w2901 = "  "
                  # "List box formatting"
                  n2539 = Build Array(w2845, w2913, w2848) -> (w2911:T3)
                  n2540 = Build Array(w2846, w2914, w2849) -> (w2912:T3)
                  n2541 = Build Array(w2843, w2844, w2915, w2850) -> (w2907:T3)
                  n2542 = Build Array (concatenate)(w2912, w2911) -> (w2910:T3)
                  n2543 = Decrement(x=w2849) -> (x-1=w2889:dbl)
                  n2544 = Decrement(x=w2850) -> (x-1=w2888:dbl)
                  n2545 = Decrement(x=w2848) -> (x-1=w2890:dbl)
                  n2546 = Multiply(x=w2889, y=w2839) -> (x*y=w2863:dbl)
                  n2547 = Multiply(x=w2888, y=w2839) -> (x*y=w2855:dbl)
                  n2548 = Multiply(x=w2890, y=w2839) -> (x*y=w2882:dbl)
                  n2549 = Build Array (concatenate)(w2909, w2910) -> (w2905:T3)
                  n2550 = Index Array(array=w2884, index (row)=w2855, index (col)=w2856) -> (element=w2885:bool)
                  n2551 = Index Array(array=w2884, index (row)=w2863, index (col)=w2864) -> (element=w2886:bool)
                  n2552 = Index Array(array=w2884, index (row)=w2882, index (col)=w2881) -> (element=w2887:bool)
                  n2553 = Index Array(array=w2847, index (row)=w2863, index (col)=w2864) -> (element=w2865:dbl)
                  n2554 = Index Array(array=w2847, index (row)=w2882, index (col)=w2881) -> (element=w2878:dbl)
                  n2555 = Index Array(array=w2847, index (row)=w2855, index (col)=w2856) -> (element=w2838:dbl)
                  n2556 = Greater Than 0?(x=w2838) -> (x > 0?=w2837:bool)
                  n2557 = Greater Than 0?(x=w2865) -> (x > 0?=w2862:bool)
                  n2558 = Greater Than 0?(x=w2878) -> (x > 0?=w2879:bool)
                  n2559 = Number To Fractional String(number=w2865, precision (6)=i16 1) -> (F-format string=w2866:string)  [unwired: 2 in]
                  n2560 = Number To Fractional String(number=w2878, precision (6)=i16 1) -> (F-format string=w2877:string)  [unwired: 2 in]
                  n2561 = Number To Fractional String(number=w2838, precision (6)=i16 1) -> (F-format string=w2860:string)  [unwired: 2 in]
                  n2562 = Concatenate Strings(w2866, " wt in hole") -> (w2861:string)
                  n2563 = Concatenate Strings(w2877, " wt in hole") -> (w2875:string)
                  n2564 = Concatenate Strings(w2860, " wt in hole") -> (w2857:string)
                  n2565 = Build Array (concatenate)(w2907, w2905) -> (w2906:T3)
                  n2566 = Select(t=w2857, s=w2837, f="  ") -> (s? t:f=w2869:string)
                  n2567 = Select(t=w2875, s=w2879, f="  ") -> (s? t:f=w2873:string)
                  n2568 = Select(t=w2861, s=w2862, f="  ") -> (s? t:f=w2871:string)
                  n2569 = Number To Fractional String(number=w2906, precision (6)=i16 3) -> (F-format string=w2904:string[][])  [unwired: 2 in]
                  n2570 = Build Array(w2901, w2901, w2901, w2901) -> (w2903:string[])
                  n2571 = Select(t=w2893, s=w2885, f=w2869) -> (s? t:f=w2896:string)
                  n2572 = Select(t=w2893, s=w2886, f=w2871) -> (s? t:f=w2895:string)
                  n2573 = Select(t=w2893, s=w2887, f=w2873) -> (s? t:f=w2894:string)
                  n2574 = Insert Into Array(array=w2904, index (row)=1, new element=w2903) -> (w2900:string[][])  [unwired: 1 in]
                  n2575 = Replace Array Subset(array=w2900, new element=w2901, index (row)=3 ("disabled index (row)"), index (col)=0 ("disabled index (col)")) -> (w2891:string[][])
                  n2576 = Build Array(w2896, "  ", w2895, w2894) -> (w2892:string[])
                  n2577 = Initialize Array("  ", w2852, w2852) -> (w2853:string[][])
                  n2578 = Insert Into Array(array=w2891, index (col)=4 ("disabled index (col)"), new element=w2892) -> (w2854:string[][])  [unwired: 1 in]
                  n2579 = property on="Fwd Generator Balance Plane Split Options" class="MCListbox (strict)"("ItemNames"=w2853) -> ()  [unwired: 2 in, 2 out]
                  n2580 = property on="Aft Generator Balance Plane Split Options" class="MCListbox (strict)"("ItemNames"=w2853) -> ()  [unwired: 2 in, 2 out]
                  n2581 = property on="Fwd Turbine Balance Plane Split Options" class="MCListbox (strict)"("ItemNames"=w2853) -> ()  [unwired: 2 in, 2 out]
                  n2582 = property on="Aft Turbine Balance Plane Split Options" class="MCListbox (strict)"("ItemNames"=w2854) -> ()  [unwired: 2 in, 2 out]
                  "AT Correction 1" <- w2842
                  "AT Correction 2A" <- w2841
                  "AT Correction 2B" <- w2840
                }
                frame 1 {
                  w2930 = 1 ("disabled index (col)")
                  w2940 = 1 ("disabled index (col)")
                  w2957 = 1 ("disabled index (col)")
                  w2969 = "Occupied!  "
                  w2977 = "  "
                  # "List box formatting"
                  n2583 = Build Array "Mass,angle, loc"(w2920, w2989, w2925) -> (w2987:T3)
                  n2584 = Build Array "Percent,mass,angle,location"(w2921, w2922, w2991, w2927) -> (w2983:T3)
                  n2585 = Build Array "Mass,angle, loc"(w2923, w2990, w2926) -> (w2988:T3)
                  n2586 = Build Array (concatenate)(w2988, w2987) -> (w2986:T3)
                  n2587 = Decrement(x=w2926) -> (x-1=w2965:dbl)
                  n2588 = Decrement(x=w2927) -> (x-1=w2964:dbl)
                  n2589 = Decrement(x=w2925) -> (x-1=w2966:dbl)
                  n2590 = Multiply(x=w2965, y=w2916) -> (x*y=w2939:dbl)
                  n2591 = Multiply(x=w2964, y=w2916) -> (x*y=w2929:dbl)
                  n2592 = Multiply(x=w2966, y=w2916) -> (x*y=w2958:dbl)
                  n2593 = Build Array (concatenate)(w2985, w2986) -> (w2981:T3)
                  n2594 = Index Array(array=w2960, index (row)=w2929, index (col)=w2930) -> (element=w2961:bool)
                  n2595 = Index Array(array=w2960, index (row)=w2939, index (col)=w2940) -> (element=w2962:bool)
                  n2596 = Index Array(array=w2960, index (row)=w2958, index (col)=w2957) -> (element=w2963:bool)
                  n2597 = Index Array(array=w2924, index (row)=w2939, index (col)=w2940) -> (element=w2941:dbl)
                  n2598 = Index Array(array=w2924, index (row)=w2958, index (col)=w2957) -> (element=w2954:dbl)
                  n2599 = Index Array(array=w2924, index (row)=w2929, index (col)=w2930) -> (element=w2936:dbl)
                  n2600 = Greater Than 0?(x=w2941) -> (x > 0?=w2938:bool)
                  n2601 = Greater Than 0?(x=w2954) -> (x > 0?=w2955:bool)
                  n2602 = Greater Than 0?(x=w2936) -> (x > 0?=w2932:bool)
                  n2603 = Number To Fractional String(number=w2941, precision (6)=i16 1) -> (F-format string=w2942:string)  [unwired: 2 in]
                  n2604 = Number To Fractional String(number=w2954, precision (6)=i16 1) -> (F-format string=w2953:string)  [unwired: 2 in]
                  n2605 = Number To Fractional String(number=w2936, precision (6)=i16 1) -> (F-format string=w2935:string)  [unwired: 2 in]
                  n2606 = Concatenate Strings(w2942, " wt in hole") -> (w2937:string)
                  n2607 = Concatenate Strings(w2953, " wt in hole") -> (w2951:string)
                  n2608 = Concatenate Strings(w2935, " wt in hole") -> (w2931:string)
                  n2609 = Build Array (concatenate)(w2983, w2981) -> (w2982:T3)
                  n2610 = Select(t=w2931, s=w2932, f="  ") -> (s? t:f=w2945:string)
                  n2611 = Select(t=w2951, s=w2955, f="  ") -> (s? t:f=w2949:string)
                  n2612 = Select(t=w2937, s=w2938, f="  ") -> (s? t:f=w2947:string)
                  n2613 = Number To Fractional String(number=w2982, precision (6)=i16 3) -> (F-format string=w2980:string[][])  [unwired: 2 in]
                  n2614 = Build Array(w2977, w2977, w2977, w2977) -> (w2979:string[])
                  n2615 = Select(t=w2969, s=w2961, f=w2945) -> (s? t:f=w2972:string)
                  n2616 = Select(t=w2969, s=w2962, f=w2947) -> (s? t:f=w2971:string)
                  n2617 = Select(t=w2969, s=w2963, f=w2949) -> (s? t:f=w2970:string)
                  n2618 = Insert Into Array(array=w2980, index (row)=1, new element=w2979) -> (w2976:string[][])  [unwired: 1 in]
                  n2619 = Replace Array Subset(array=w2976, new element=w2977, index (row)=3 ("disabled index (row)"), index (col)=0 ("disabled index (col)")) -> (w2967:string[][])
                  n2620 = Build Array(w2972, "  ", w2971, w2970) -> (w2968:string[])
                  n2621 = Insert Into Array(array=w2967, index (col)=4 ("disabled index (col)"), new element=w2968) -> (w2928:string[][])  [unwired: 1 in]
                  n2622 = property on="Fwd Turbine Balance Plane Split Options" class="MCListbox (strict)"("ItemNames"=w2928) -> ()  [unwired: 2 in, 2 out]
                  "FT Correction 1" <- w2919
                  "FT Correction 2A" <- w2918
                  "FT Correction 2B" <- w2917
                }
                frame 2 {
                  w3005 = 2 ("disabled index (col)")
                  w3015 = 2 ("disabled index (col)")
                  w3032 = 2 ("disabled index (col)")
                  w3044 = "Occupied!  "
                  w3052 = "  "
                  # "List box formatting"
                  n2623 = Build Array "Mass,angle, loc"(w2998, w3064, w3000) -> (w3062:T3)
                  n2624 = Build Array "Mass,angle, loc"(w2997, w3065, w3001) -> (w3063:T3)
                  n2625 = Build Array "Percent,mass,angle,location"(w3066, w2996, w3067, w3002) -> (w3058:T3)
                  n2626 = Build Array (concatenate)(w3063, w3062) -> (w3061:T3)
                  n2627 = Decrement(x=w3001) -> (x-1=w3040:dbl)
                  n2628 = Decrement(x=w3002) -> (x-1=w3039:dbl)
                  n2629 = Decrement(x=w3000) -> (x-1=w3041:dbl)
                  n2630 = Multiply(x=w3040, y=w2992) -> (x*y=w3014:dbl)
                  n2631 = Multiply(x=w3039, y=w2992) -> (x*y=w3004:dbl)
                  n2632 = Multiply(x=w3041, y=w2992) -> (x*y=w3033:dbl)
                  n2633 = Build Array (concatenate)(w3060, w3061) -> (w3056:T3)
                  n2634 = Index Array(array=w3035, index (row)=w3004, index (col)=w3005) -> (element=w3036:bool)
                  n2635 = Index Array(array=w3035, index (row)=w3014, index (col)=w3015) -> (element=w3037:bool)
                  n2636 = Index Array(array=w3035, index (row)=w3033, index (col)=w3032) -> (element=w3038:bool)
                  n2637 = Index Array(array=w2999, index (row)=w3014, index (col)=w3015) -> (element=w3016:dbl)
                  n2638 = Index Array(array=w2999, index (row)=w3033, index (col)=w3032) -> (element=w3029:dbl)
                  n2639 = Index Array(array=w2999, index (row)=w3004, index (col)=w3005) -> (element=w3011:dbl)
                  n2640 = Greater Than 0?(x=w3016) -> (x > 0?=w3013:bool)
                  n2641 = Greater Than 0?(x=w3029) -> (x > 0?=w3030:bool)
                  n2642 = Greater Than 0?(x=w3011) -> (x > 0?=w3007:bool)
                  n2643 = Number To Fractional String(number=w3016, precision (6)=i16 1) -> (F-format string=w3017:string)  [unwired: 2 in]
                  n2644 = Number To Fractional String(number=w3029, precision (6)=i16 1) -> (F-format string=w3028:string)  [unwired: 2 in]
                  n2645 = Number To Fractional String(number=w3011, precision (6)=i16 1) -> (F-format string=w3010:string)  [unwired: 2 in]
                  n2646 = Concatenate Strings(w3017, " wt in hole") -> (w3012:string)
                  n2647 = Concatenate Strings(w3028, " wt in hole") -> (w3026:string)
                  n2648 = Concatenate Strings(w3010, " wt in hole") -> (w3006:string)
                  n2649 = Build Array (concatenate)(w3058, w3056) -> (w3057:T3)
                  n2650 = Select(t=w3006, s=w3007, f="  ") -> (s? t:f=w3020:string)
                  n2651 = Select(t=w3026, s=w3030, f="  ") -> (s? t:f=w3024:string)
